vi "King Danger after Swap.vi"(9 "Cell to Swap":i32, 10 "DT Team #":i32, 11 "1D Board":T1[](array[typedef])) -> (3 "King in Danger?":bool)   [LabVIEW 2014]
uses:
  Typedefs/Board Cell.ctl
  Typedefs/Cell Occupancy.ctl
  Dragon Tamers.lvlib
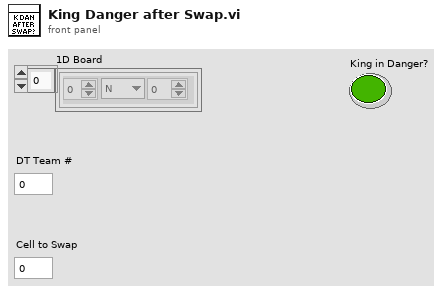
[diagram p1: front panel]
types:
  T1 = typedef "Dragon Tamers.lvlib/Board Cell.ctl" = cluster{"Team":i32, "Occu.":T2, "Count":i32}
  T2 = typedef "Dragon Tamers.lvlib/Cell Occupancy.ctl" = enum16{"N", "C", "K"}
  T3 = typedef "Dragon Tamers.lvlib/Parsed Board.ctl" = cluster{"DT King":i32, "Opp King":i32, "Count":i32[], "Empty Cells":i32[], "DT Cells":i32[], "Opp Cells":i32[], "DT Team":i32, "Opp. Team":i32}
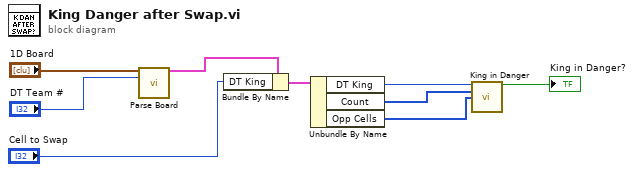
[diagram p0: block diagram]
diagram:
  n1 = call "Parse Board.vi"("Board Array"="1D Board", "DT Team #"="DT Team #") -> ("Parsed Board Info"=w7:T3)  [unwired: 12 in, 1 out]
  n2 = Bundle By Name(cluster=w7, "DT King"="Cell to Swap") -> (w5:T3)
  n3 = Unbundle By Name(w5) -> ("DT King"=w4:i32, "Count"=w3:i32[], "Opp Cells"=w2:i32[])
  n4 = call "King in Danger.vi"("King Index"=w4, "Count"=w3, "Opp Team Cells"=w2) -> ("King in Danger?"=→"King in Danger?":bool)  [unwired: 9 in, 3 out]
